vi "Endpoint Connected.vi"(8 "error in":errorcluster, 10 "Endpoint":refnum<class "Message Enqueuer.lvclass">, 11 "Target Reply Time Test Actor in":refnum<class "Target Reply Time Test Actor.lvclass">) -> (0 "error out":errorcluster, 3 "Target Reply Time Test Actor out":refnum<class "Target Reply Time Test Actor.lvclass">)   [LabVIEW 2023, in "Target Reply Time Test Actor.lvlib" / "Target Reply Time Test Actor.lvclass"]
doc: "Override this method to specify how the receiving actor responds to a Connected message from a nested endpoint actor."
uses:
  <vilib>/ActorFramework/Message Enqueuer/Message Enqueuer.lvclass
  Target Reply Time Test Actor.lvclass
  Target Reply Time Test Actor.lvclass/Target Reply Time Test Actor.ctl
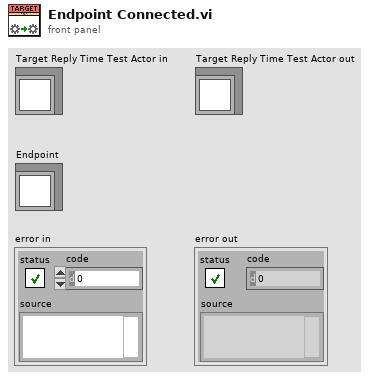
[diagram p1: front panel]
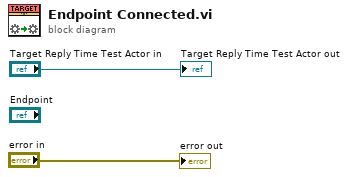
[diagram p0: block diagram]
diagram:
  "error out" <- "error in"
  "Target Reply Time Test Actor out" <- "Target Reply Time Test Actor in"
